vi "Parse Record Items By Name.vi"(9 "Record Names":string[](array[string]), 10 "header map in":map{string, i32}(c390), 11 "Record in":string[](array[string])) -> (0 "found all":bool, 1 "Values":string[](array[string]), 2 "header map out":map{string, i32}(c390), 3 "Record out":string[](array[string]))   [LabVIEW 2020, in "Configuration_Helper.lvlib"]
uses:
  Configuration_Helper.lvlib
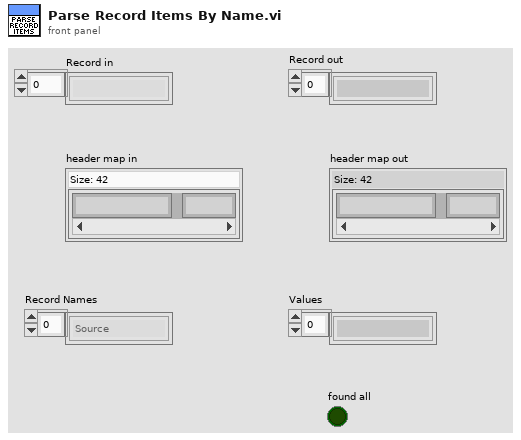
[diagram p1: front panel]
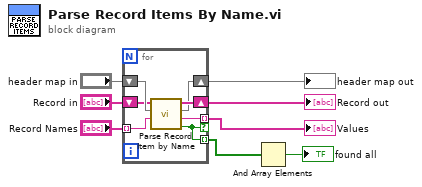
[diagram p0: block diagram]
diagram:
  n1 = for {
    shift-right: [w12] -> w5
    shift-left: "Record in" -> [w13]
    tunnel: "Record Names" -> [w14] mode=indexing
    shift-right: [w10] -> w4
    shift-left: "header map in" -> [w15]
    tunnel: [w11] -> w3 mode=indexing if=w9
    tunnel: [w9] -> w2 mode=indexing
    n2 = call "Parse Record Item by Name.vi"("key"=w14, "header map in"=w15, "Record in in"=w13) -> ("found"=w9:bool, "Value"=w11:string, "header map out"=w10:map{string, i32}, "Record out"=w12:string[])  [unwired: 5 in]
  }
  "Record out" <- w5
  "header map out" <- w4
  "Values" <- w3
  n3 = And Array Elements(Boolean array=w2) -> (logical AND=→"found all":bool)
